vi "Get Count.vi"(8 "error in (no error)":errorcluster, 11 "Core Groups Configuration in":refnum<class "Core Groups Configuration.lvclass">) -> (0 "error out":errorcluster, 2 "count":i32, 3 "Core Groups Configuration out":refnum<class "Core Groups Configuration.lvclass">)   [LabVIEW 2017, in "DSF Core.lvlib" / "Core Groups Configuration.lvclass"]
uses:
  Core Groups Configuration.lvclass
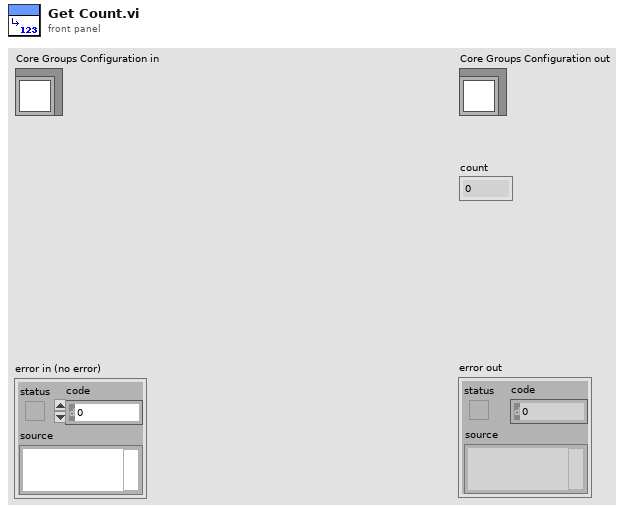
[diagram p1: front panel]
types:
  T1 = typedef "DSF Core.lvlib/Core Groups Configuration.lvclass/Configuration.ctl" = cluster{"name":string, "direction":T2, "cycle timing":T3, "timeout behavior":T4, "convert buffers":bool}
  T2 = typedef "DSF Core.lvlib/DSF Direction.ctl" = enum8{"Tx", "Rx"}
  T3 = typedef "DSF Core.lvlib/DSF Timing Info.ctl" = cluster{"priority":u64, "decimation":u64, "offset":u64}
  T4 = typedef "DSF Core.lvlib/DSF Timeout Behavior.ctl" = enum8{"Increment Late Count", "Throw Error"}
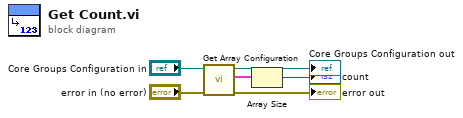
[diagram p0: block diagram]
diagram:
  n1 = call "Get Array Configuration.vi"("error in (no error)"="error in (no error)", "Core Groups Configuration in"="Core Groups Configuration in") -> ("error out"=→"error out":errorcluster, "group configurations"=w2:T1[], "Core Groups Configuration out"=→"Core Groups Configuration out":refnum<class "Core Groups Configuration.lvclass">)  [unwired: 7 in]
  n2 = Array Size(array=w2) -> (size(s)=→"count":i32)
